vi "Read NMEA GPS SubVI.vi"(0 "VISA resource name":refnum<visa-resource-name>="COM1", 1 "timeout (ms)":u32=10000, 2 "UTC Time Zone":i32, 3 "error in (no error)":errorcluster, 4 "stop":bool) -> (5 "GPS Data":T1 {"Course over ground (degrees)" format="%#.6g"; "Speed over ground (knots)" format="%#.6g"; "Magnetic Variation (degrees)" format="%#.6g"; "Longitude (ddmm.mmmm)" format="%#.6g"; "Lattitude (ddmm.mmmm)" format="%#.6g"}, 6 "GPS Data Valid?":bool, 7 "error out":errorcluster)   [LabVIEW 2010]
doc: "This subVI decodes the most common NMEA-0183 sentence transmitted by GPS receivers, the $GPRMC sentence. The subvi returns time, position, ground speed, and magnetic variation. In the GPS interface configuration, use the \"NMEA OUT\" setting and set the baud rate to the standard 4800 bps setting. Connected to the computer's serial port using a PC Interface Cable, available from the GPS vendor. This subvi initializes the serial port on first call. On subsequent calls, the initialization is skipped. Always use the Stop input when stopping the VI so that the serial port connection is closed."
uses:
  <vilib>/Instr/_visa.llb/VISA Configure Serial Port (Instr).vi
panel:
  in  "Cluster":T1 {"Course over ground (degrees)" format="%_4g"; "Speed over ground (knots)" format="%_3g"; "Magnetic Variation (degrees)" format="%_4g"; "Longitude (ddmm.mmmm)" format="%_8g"; "Lattitude (ddmm.mmmm)" format="%_8g"}
  out "Variation East/West":string
  out "Magnetic Variation (degrees)":dbl format="%_4g"
  out "Course over ground (degrees)":dbl format="%_4g"
  out "Speed over ground (knots)":dbl format="%_3g"
  out "Longitude East/West":string
  out "Longitude (ddmm.mmmm)":dbl format="%_8g"
  out "Lattitude North/South":string
  out "Lattitude (ddmm.mmmm)":dbl format="%_8g"
  out "Local Time":timestamp
  out "UTC Time":timestamp
  in  "date time rec":T2
  out "Bytes read":u32
  out "String Read":string="\n"
  # "This subVI decodes the most common NMEA-0183 sentence transmitted by GPS receivers, the $GPRMC sentence. The subvi returns time, position, ground speed, and magnetic variation. In the GPS interface configuration, use the \"NMEA OUT\" setting and set the baud rate to the standard 4800 bps setting. Connected to the computer's serial port using a PC Interface Cable, available from the GPS vendor. This subvi initializes the serial port on first call. On subsequent calls, the initialization is skipped. Always use the Stop input when stopping the VI so that the serial port connection is closed."
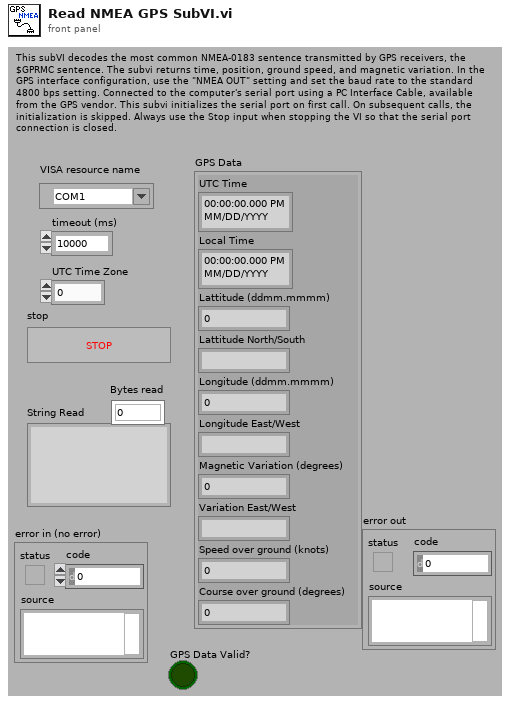
[diagram p1: front panel]
types:
  T1 = cluster{"UTC Time":timestamp, "Local Time":timestamp, "Lattitude (ddmm.mmmm)":dbl, "Lattitude North/South":string, "Longitude (ddmm.mmmm)":dbl, "Longitude East/West":string, "Magnetic Variation (degrees)":dbl, "Variation East/West":string, "Speed over ground (knots)":dbl, "Course over ground (degrees)":dbl}
  T2 = cluster{"second":i32, "minute":i32, "hour":i32, "day of month":i32, "month":i32, "year":i32, "day of week":i32, "day of year":i32, "is DST":i32}
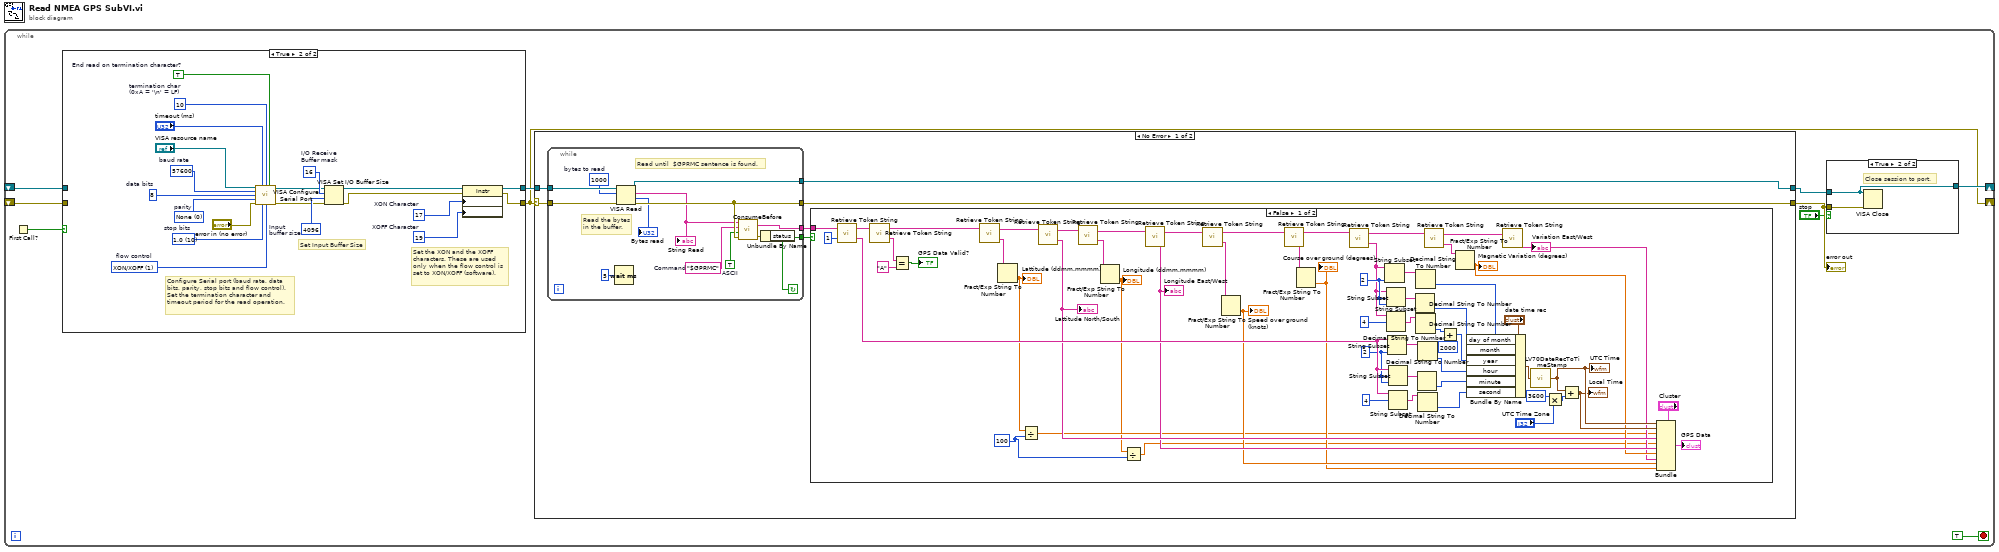
[diagram p0: block diagram]
diagram:
  n1 = while {
    shift-right: [w6] -> _
    shift-left: _ -> [w5]
    shift-right: [w4] -> _
    shift-left: _ -> [w3]
    stop <- TRUE stop-if-true
    n2 = First Call?() -> (First Call?: T/F=w8:bool)
    n3 = case shown="True" w8 {
      tunnel: [w15 w20] -> w10
      tunnel: [w14 w17] -> w4
      tunnel: w5 -> [w15 _]
      tunnel: w3 -> [w14 _]
      frame False {
      }
      frame True {
        w30 = TRUE  # End read on termination character?
        w22 = u8 19  # XOFF Character
        w23 = u8 17  # XON Character
        w28 = u32 4096  # Input buffer size
        w26 = u16 1 items=["None"=0, "XON/XOFF"=1, "RTS/CTS"=2, "DTR/DSR"=4]  # flow control
        w32 = u16 10 items=["1.0"=10, "1.5"=15, "2.0"=20]  # stop bits
        w33 = u16 0 items=["None", "Odd", "Even", "Mark", "Space"]  # parity
        w21 = u16 8  # data bits
        w35 = u32 57600  # baud rate
        w27 = u8 10  # termination char (0xA = '\n' = LF)
        w29 = u16 16  # I/O Receive Buffer mask
        # "Set the XON and the XOFF\ncharacters. These are used\nonly when the flow control is\nset to XON/XOFF (software)."
        # "Configure Serial port (baud rate, data\nbits, parity, stop bits and flow control).\nSet the termination character and\ntimeout period for the read operation."
        # "Set Input Buffer Size"
        n4 = call-poly "VISA Configure Serial Port"("VISA resource name"="VISA resource name", "timeout (10sec)"="timeout (ms)", "termination char\n(0xA = '\\n' = LF)"=w27, "Enable Termination\nChar (T)"=w30, "baud rate (9600)"=w35, "data bits (8)"=w21, "parity (0:none)"=w33, "error in (no error)"="error in (no error)", "stop bits (10: 1 bit)"=w32, "flow control (0:none)"=w26) -> ("VISA resource name out"=w19:refnum<visa-resource-name>, "error out"=w18:errorcluster)  [unwired: 4 in]
        n5 = VISA Set I/O Buffer Size(VISA resource name=w19, mask (16)=w29, size (4096)=w28, error in (no error)=w18) -> (VISA resource name out=w25:refnum<visa-resource-name>, error out=w24:errorcluster)
        n6 = property class="Instr"(reference=w25, error in=w24, "Serial Settings:Flow Control XON Character"=w23, "Serial Settings:Flow Control XOFF Character"=w22) -> (reference out=w20:refnum<visa-resource-name>, error out=w17:errorcluster)
      }
    }
    n7 = case shown="No Error" w4 {
      selector: w4 -> [w38 w115]
      tunnel: w10 -> [w41 w116]
      tunnel: [w40 w116] -> w9
      tunnel: [w39 w115] -> w2
      frame No Error {
        n8 = while {
          tunnel: w41 -> [w54]
          tunnel: [w53] -> w40
          tunnel: [w52] -> w39
          tunnel: w38 -> [w51]
          tunnel: [w47] -> w37
          tunnel: [w43] -> w36
          stop <- w43 continue-if-true
          w45 = u32 1000  # bytes to read
          w50 = "$GPRMC"  # Command
          w49 = TRUE  # ASCII
          # "Read until  $GPRMC sentence is found."
          # "Read the bytes\nin the buffer."
          n9 = Wait (ms)(milliseconds to wait=u32 5 ("millisecond multiple")) -> ()  [unwired: 1 out]
          n10 = VISA Read(VISA resource name=w54, byte count=w45, error in (no error)=w51) -> (VISA resource name out=w53:refnum<visa-resource-name>, read buffer=w48:string, return count=→"Bytes read":u32, error out=w52:errorcluster)
          "String Read" <- w48
          n11 = call "ConsumeBefore.vi"("error in"=w52, "ASCII"=w49, "Before"=w50, "Response String In"=w48) -> ("error out"=w46:errorcluster, "Response String Out"=w47:string)
          n12 = Unbundle By Name(w46) -> ("status"=w43:bool)
        }
        n13 = case shown="False" w36 {
          tunnel: w37 -> [w112 _]
          frame False {
            w55 = 100
            w80 = 2 ("length (rest)")
            w102 = 2 ("length (rest)")
            n14 = call "Retrieve Token String.vi"("Offset (0)"=1, "input string"=w112) -> ("token string"=w109:string, "output string"=w110:string)
            n15 = call "Retrieve Token String.vi"("input string"=w110) -> ("token string"=w114:string, "output string"=w108:string)  [unwired: 1 in]
            n16 = Equal?(x=w114, y="A") -> (x = y?=→"GPS Data Valid?":bool)
            n17 = call "Retrieve Token String.vi"("input string"=w108) -> ("token string"=w93:string, "output string"=w92:string)  [unwired: 1 in]
            n18 = Fract/Exp String To Number(string=w93) -> (number=w59:dbl)  [unwired: 3 in, 1 out]
            "Lattitude (ddmm.mmmm)" <- w59
            n19 = Divide(x=w59, y=w55) -> (x/y=w58:dbl)
            n20 = call "Retrieve Token String.vi"("input string"=w92) -> ("token string"=w67:string, "output string"=w91:string)  [unwired: 1 in]
            "Lattitude North/South" <- w67
            n21 = call "Retrieve Token String.vi"("input string"=w91) -> ("token string"=w90:string, "output string"=w89:string)  [unwired: 1 in]
            n22 = Fract/Exp String To Number(string=w90) -> (number=w57:dbl)  [unwired: 3 in, 1 out]
            "Longitude (ddmm.mmmm)" <- w57
            n23 = Divide(x=w57, y=w55) -> (x/y=w56:dbl)
            n24 = call "Retrieve Token String.vi"("input string"=w89) -> ("token string"=w66:string, "output string"=w88:string)  [unwired: 1 in]
            "Longitude East/West" <- w66
            n25 = call "Retrieve Token String.vi"("input string"=w88) -> ("token string"=w87:string, "output string"=w86:string)  [unwired: 1 in]
            n26 = Fract/Exp String To Number(string=w87) -> (number=w63:dbl)  [unwired: 3 in, 1 out]
            "Speed over ground (knots)" <- w63
            n27 = call "Retrieve Token String.vi"("input string"=w86) -> ("token string"=w85:string, "output string"=w84:string)  [unwired: 1 in]
            n28 = Fract/Exp String To Number(string=w85) -> (number=w62:dbl)  [unwired: 3 in, 1 out]
            "Course over ground (degrees)" <- w62
            n29 = call "Retrieve Token String.vi"("input string"=w84) -> ("token string"=w78:string, "output string"=w72:string)  [unwired: 1 in]
            n30 = String Subset(string=w78, length (rest)=w80) -> (substring=w79:string)  [unwired: 1 in]
            n31 = String Subset(string=w78, offset (0)=w80, length (rest)=w80) -> (substring=w81:string)
            n32 = String Subset(string=w78, offset (0)=4) -> (substring=w83:string)  [unwired: 1 in]
            n33 = String Subset(string=w109, length (rest)=w102) -> (substring=w106:string)  [unwired: 1 in]
            n34 = String Subset(string=w109, offset (0)=w102, length (rest)=w102) -> (substring=w100:string)
            n35 = String Subset(string=w109, offset (0)=4) -> (substring=w98:string)  [unwired: 1 in]
            n36 = Decimal String To Number(string=w81) -> (number=w76:i32)  [unwired: 2 in, 1 out]
            n37 = Decimal String To Number(string=w79) -> (number=w77:i32)  [unwired: 2 in, 1 out]
            n38 = Decimal String To Number(string=w83) -> (number=w75:i32)  [unwired: 2 in, 1 out]
            n39 = Decimal String To Number(string=w100) -> (number=w101:i32)  [unwired: 2 in, 1 out]
            n40 = Decimal String To Number(string=w106) -> (number=w103:i32)  [unwired: 2 in, 1 out]
            n41 = Decimal String To Number(string=w98) -> (number=w97:i32)  [unwired: 2 in, 1 out]
            n42 = call "Retrieve Token String.vi"("input string"=w72) -> ("token string"=w71:string, "output string"=w70:string)  [unwired: 1 in]
            n43 = Add(x=w75, y=2000) -> (x+y=w73:i32)
            n44 = Fract/Exp String To Number(string=w71) -> (number=w65:dbl)  [unwired: 3 in, 1 out]
            "Magnetic Variation (degrees)" <- w65
            n45 = Bundle By Name(cluster="date time rec", "day of month"=w77, "month"=w76, "year"=w73, "hour"=w103, "minute"=w101, "second"=w97) -> (w105:T2)
            n46 = call "Retrieve Token String.vi"("input string"=w70) -> ("token string"=w64:string)  [unwired: 1 in, 1 out]
            "Variation East/West" <- w64
            n47 = call <vilib>:"LV70DateRecToTimeStamp.vi"("date time rec"=w105) -> ("Time Stamp"=w69:timestamp)
            "UTC Time" <- w69
            n48 = Multiply(x=3600 ("number"), y="UTC Time Zone") -> (x*y=w94:i32)
            n49 = Add(x=w69, y=w94) -> (x+y=w68:timestamp)
            "Local Time" <- w68
            n50 = Bundle(cluster="Cluster", "UTC Time"=w69, "Local Time"=w68, "Lattitude (ddmm.mmmm)"=w58, "Lattitude North/South"=w67, "Longitude (ddmm.mmmm)"=w56, "Longitude East/West"=w66, "Magnetic Variation (degrees)"=w65, "Variation East/West"=w64, "Speed over ground (knots)"=w63, "Course over ground (degrees)"=w62) -> (→"GPS Data":T1)
          }
          frame True {
          }
        }
      }
      frame Error {
      }
    }
    "error out" <- w2
    n51 = case shown="True" "stop" {
      tunnel: w9 -> [w11 w12]
      tunnel: w2 -> [_ w13]
      tunnel: [w11 w12] -> w6
      frame False {
      }
      frame True {
        # "Close session to port."
        n52 = VISA Close(VISA resource name=w12, error in (no error)=w13) -> ()  [unwired: 1 out]
      }
    }
  }
